vi "Example Error.vi"() -> ()   [LabVIEW 2013, in "Stanford Research CG635.lvlib"]
uses:
  <instrlib>/Stanford Research CG635/Stanford Research CG635.lvlib
panel:
  in  "VISA resource name":refnum<visa-resource-name>
  in  "Q / Q  Level (0: ECL)":u16(ring) items=["ECL Levels (-1.00/-1.80 V)", "+7 dBm Levels (+0.50/-0.50 V)", "LVDS Levels (1.43/1.07 V)", "PECL 3.3 V Levels (2.30/1.50 V)", "PECL 5.0 V Levels (4.00/3.20 V)", ""]
  in  "CMOS Level (0: 1.2V)":u16(ring) items=["1.2 V", "1.8 V", "2.5 V", "3.3 V", "5.0 V"]
  in  "Unit (1:MHz)":u16(ring)=1 items=["GHz", "MHz", "KHz", "Hz"]
  in  "Frequency (10)":dbl=10.0
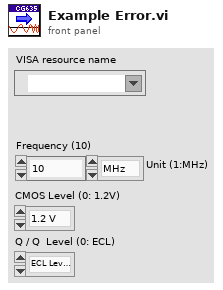
[diagram p1: front panel]
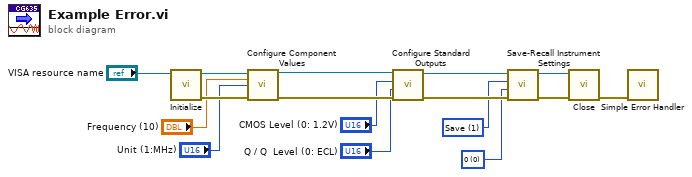
[diagram p0: block diagram]
diagram:
  w5 = u16 0 items=["0", "1", "2", "3", "4", "5", "6", "7"] ("Save Number (0)")
  w6 = u16 1 items=["Recall", "Save"] ("Recall or Save (0:Recall)")
  n1 = call <instrlib>:"Initialize.vi"("VISA resource name"="VISA resource name") -> ("error out"=w15:errorcluster, "VISA resource name out"=w16:refnum<visa-resource-name>)  [unwired: 9 in]
  n2 = call <instrlib>:"Configure Component Values.vi"("VISA resource name"=w16, "Frequency (10)"="Frequency (10)", "Unit (1:MHz)"="Unit (1:MHz)", "error in (no error)"=w15) -> ("VISA resource name out"=w12:refnum<visa-resource-name>, "error out"=w11:errorcluster)  [unwired: 10 in]
  n3 = call <instrlib>:"Configure Standard Outputs.vi"("error in (no error)"=w11, "Q / Q  Level (0: ECL)"="Q / Q  Level (0: ECL)", "CMOS Level (0: 1.2V)"="CMOS Level (0: 1.2V)", "VISA resource name"=w12) -> ("error out"=w7:errorcluster, "VISA resource name out"=w8:refnum<visa-resource-name>)  [unwired: 6 in]
  n4 = call <instrlib>:"Save-Recall Instrument Settings.vi"("error in (no error)"=w7, "Save Number (0)"=w5, "Recall or Save (0:Recall)"=w6, "VISA resource name"=w8) -> ("error out"=w3:errorcluster, "VISA resource name out"=w4:refnum<visa-resource-name>)  [unwired: 6 in]
  n5 = call <instrlib>:"Close.vi"("error in (no error)"=w3, "VISA resource name"=w4) -> ("error out"=w2:errorcluster)  [unwired: 9 in]
  n6 = call <vilib>:"Simple Error Handler.vi"("error in (no error)"=w2) -> ()  [unwired: 4 in, 5 out]
